vi "open client handle.vi"(8 "error in (no error)":errorcluster, 9 "Headers":cluster{"header":string, "value":string}[](array[cluster]), 10 "Request URI in":string, 11 "Oauth2 in":refnum<class "Oauth2.lvclass">) -> (0 "error out":errorcluster, 2 "Request URI dup":string, 3 "Oauth2 out":refnum<class "Oauth2.lvclass">)   [LabVIEW 2020, in "Oauth2.lvclass"]
uses:
  Oauth2.lvclass
  Oauth2.lvclass/Oauth2.ctl
  OauthClient/OAuthClient.lvclass
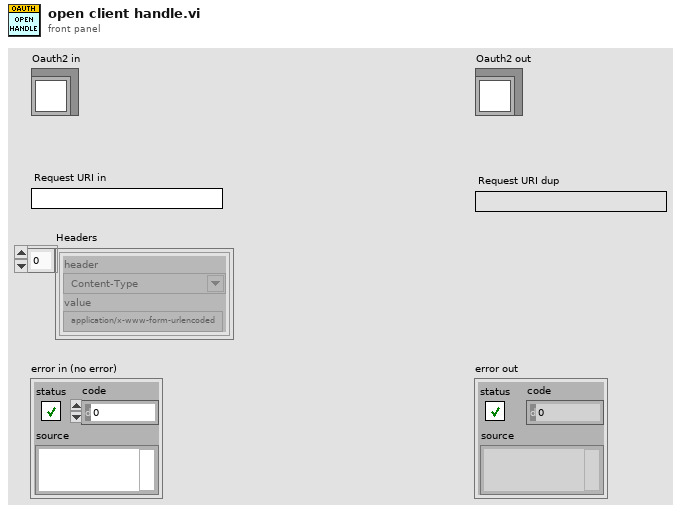
[diagram p1: front panel]
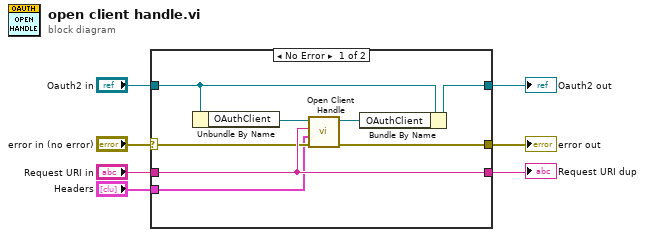
[diagram p0: block diagram]
diagram:
  n1 = case shown="No Error" "error in (no error)" {
    selector: "error in (no error)" -> [w13 w18]
    tunnel: [w12 w18] -> w6
    tunnel: [w9 w17] -> w4
    tunnel: "Oauth2 in" -> [w10 w17]
    tunnel: [w14 w16] -> w3
    tunnel: "Request URI in" -> [w14 w16]
    tunnel: "Headers" -> [w8 _]
    frame No Error {
      n2 = Unbundle By Name(w10) -> ("OAuthClient"=w15:refnum<class "OAuthClient.lvclass">)
      n3 = call-dynamic "Open Client Handle.vi"("error in (no error)"=w13, "Headers"=w8, "Request URI"=w14, "OAuthClient in"=w15) -> ("error out"=w12:errorcluster, "OAuthClient out"=w11:refnum<class "OAuthClient.lvclass">)  [unwired: 6 in]
      n4 = Bundle By Name(cluster=w10, "OAuthClient"=w11) -> (w9:refnum<class "Oauth2.lvclass">)
    }
    frame Error {
    }
  }
  "error out" <- w6
  "Oauth2 out" <- w4
  "Request URI dup" <- w3
